vi "pulse_generator_multiheater_continuous_refnum.vi"(2 "Stop! Refnum":refnum<vi>, 3 "Pulse Generator Control Multiheater Refnums":T1) -> ()   [LabVIEW 2017]
uses:
  pulse_generator_controls_multiheater_refnums.ctl
  <vilib>/Utility/error.llb/DialogType.ctl
  <vilib>/DAQmx/write.llb/DAQmx Write (Digital 1D Bool NChan 1Samp 1Line).vi
  <vilib>/DAQmx/write.llb/DAQmx Write (Digital Wfm 1Chan NSamp).vi
  <vilib>/DAQmx/write.llb/DAQmx Write (Counter 1D Frequency 1Chan NSamp).vi
  <vilib>/DAQmx/read.llb/DAQmx Read (Counter DBL 1Chan 1Samp).vi
  <extravilib>/ChannelInstances/Stream-bool/Read With Abort.vi
  <extravilib>/ChannelInstances/Stream-bool/Write With Abort.vi
  <extravilib>/ChannelInstances/Stream-bool/EndpointRead.vi
  <extravilib>/ChannelInstances/Stream-bool/Endpoint.vi
  <vilib>/DAQmx/create/channels.llb/DAQmx Create Channel (CI-Position-Angular Encoder).vi
  <vilib>/DAQmx/create/channels.llb/DAQmx Create Channel (DO-Digital Output).vi
  <vilib>/DAQmx/configure/timing.llb/DAQmx Timing (Sample Clock).vi
  <vilib>/DAQmx/create/channels.llb/DAQmx Create Channel (CO-Pulse Generation-Frequency).vi
  <vilib>/DAQmx/configure/timing.llb/DAQmx Timing (Implicit).vi
  <vilib>/DAQmx/configure/trigger.llb/DAQmx Start Trigger (Digital Edge).vi
  <vilib>/Waveform/DWDTOps.llb/DWDT Uncompress Digital.vi
  <vilib>/DAQmx/miscellaneous.llb/DAQmx Fill In Error Info.vi
  <extravilib>/ChannelInstances/Stream-bool/Instantiate.vi
  <extravilib>/ChannelInstances/Stream-bool/)Channel.vi
  <resource>/ChannelSupport/_ChannelSupport/WaitIfNeeded.vi
  <extravilib>/ChannelInstances/Stream-bool.lvlib
  <resource>/objmgr/daqmx.rc
panel:
  out "Waveform Chart":dbl(graph)
  out "Stopped!":bool caption="OK"
  in  "Stop! Local":bool
  out "message":string
  in  "SwitchHelper":bool
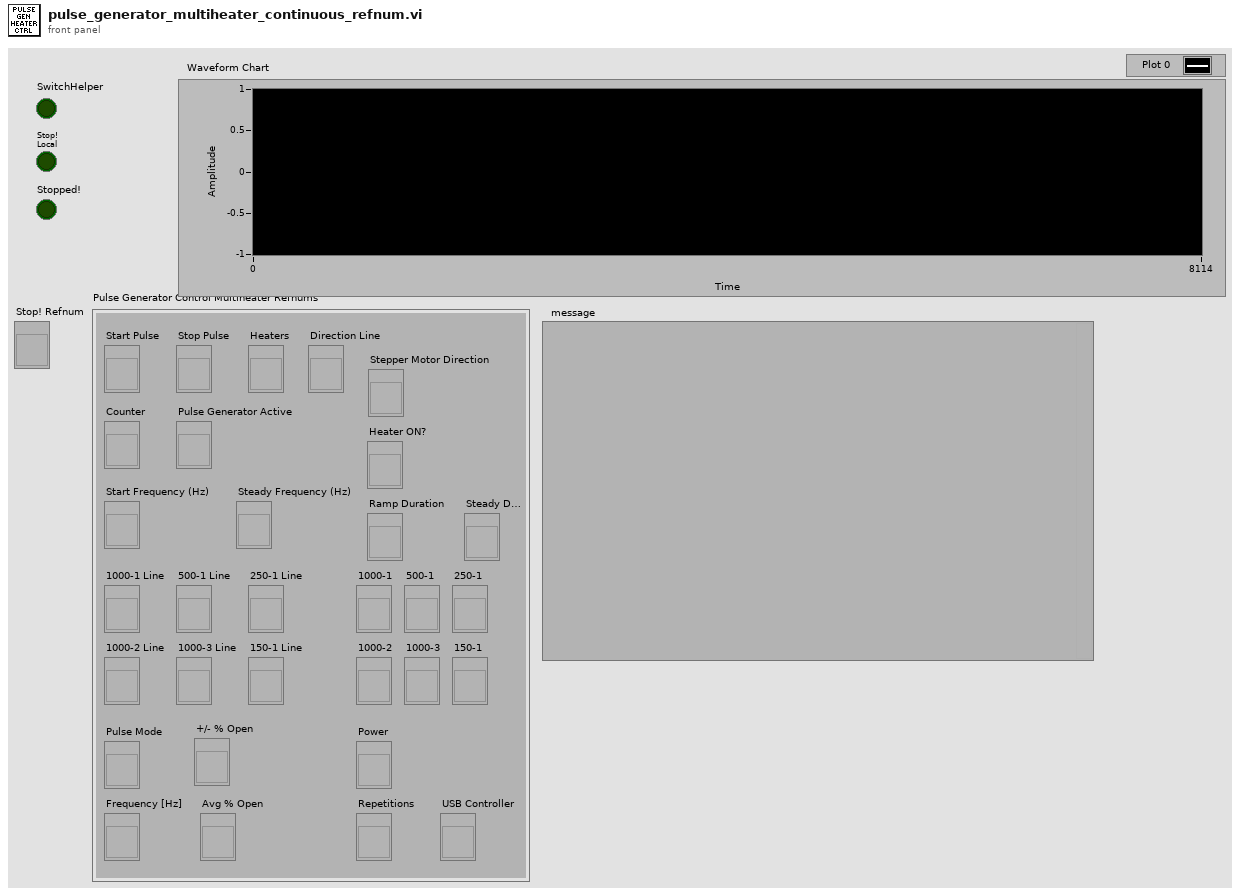
[diagram p1: front panel]
types:
  T1 = typedef "pulse_generator_controls_multiheater_refnums.ctl" = cluster{"Start Pulse":refnum<vi>, "Stop Pulse":refnum<vi>, "Heaters":refnum<vi>, "Counter":refnum<vi>, "Start Frequency (Hz)":refnum<vi>, "Pulse Generator Active":refnum<vi>, "Stepper Motor Direction":refnum<vi>, "Ramp Duration":refnum<vi>, "Direction Line":refnum<vi>, "1000-1 Line":refnum<vi>, "1000-2 Line":refnum<vi>, "1000-3 Line":refnum<vi>, "500-1 Line":refnum<vi>, "250-1 Line":refnum<vi>, "1000-1":refnum<vi>, "1000-2":refnum<vi>, "1000-3":refnum<vi>, "500-1":refnum<vi>, "250-1":refnum<vi>, "150-1":refnum<vi>, "Heater ON?":refnum<vi>, "150-1 Line":refnum<vi>, "Power":refnum<vi>, "Steady Frequency (Hz)":refnum<vi>, "Steady Duration ":refnum<vi>, "Pulse Mode":refnum<vi>, "Frequency [Hz]":refnum<vi>, "Avg % Open":refnum<vi>, "Repetitions":refnum<vi>, "+/- % Open":refnum<vi>, "USB Controller":refnum<vi>}
  T2 = enum8{"Enabled", "Disabled", "Disabled and Grayed Out"}
  T3 = typedef "DialogType.ctl" = u16
  T4 = cluster{"1000-1":refnum<vi>, "1000-2":refnum<vi>, "1000-3":refnum<vi>, "500-1":refnum<vi>, "250-1":refnum<vi>, "150-1":refnum<vi>}
  T5 = cluster{"1000-1 Line":refnum<vi>, "1000-2 Line":refnum<vi>, "1000-3 Line":refnum<vi>, "500-1 Line":refnum<vi>, "250-1 Line":refnum<vi>, "150-1 Line":refnum<vi>}
  T6 = typedef "Stream-bool.lvlib/)Channel.ctl" = refnum<queue>
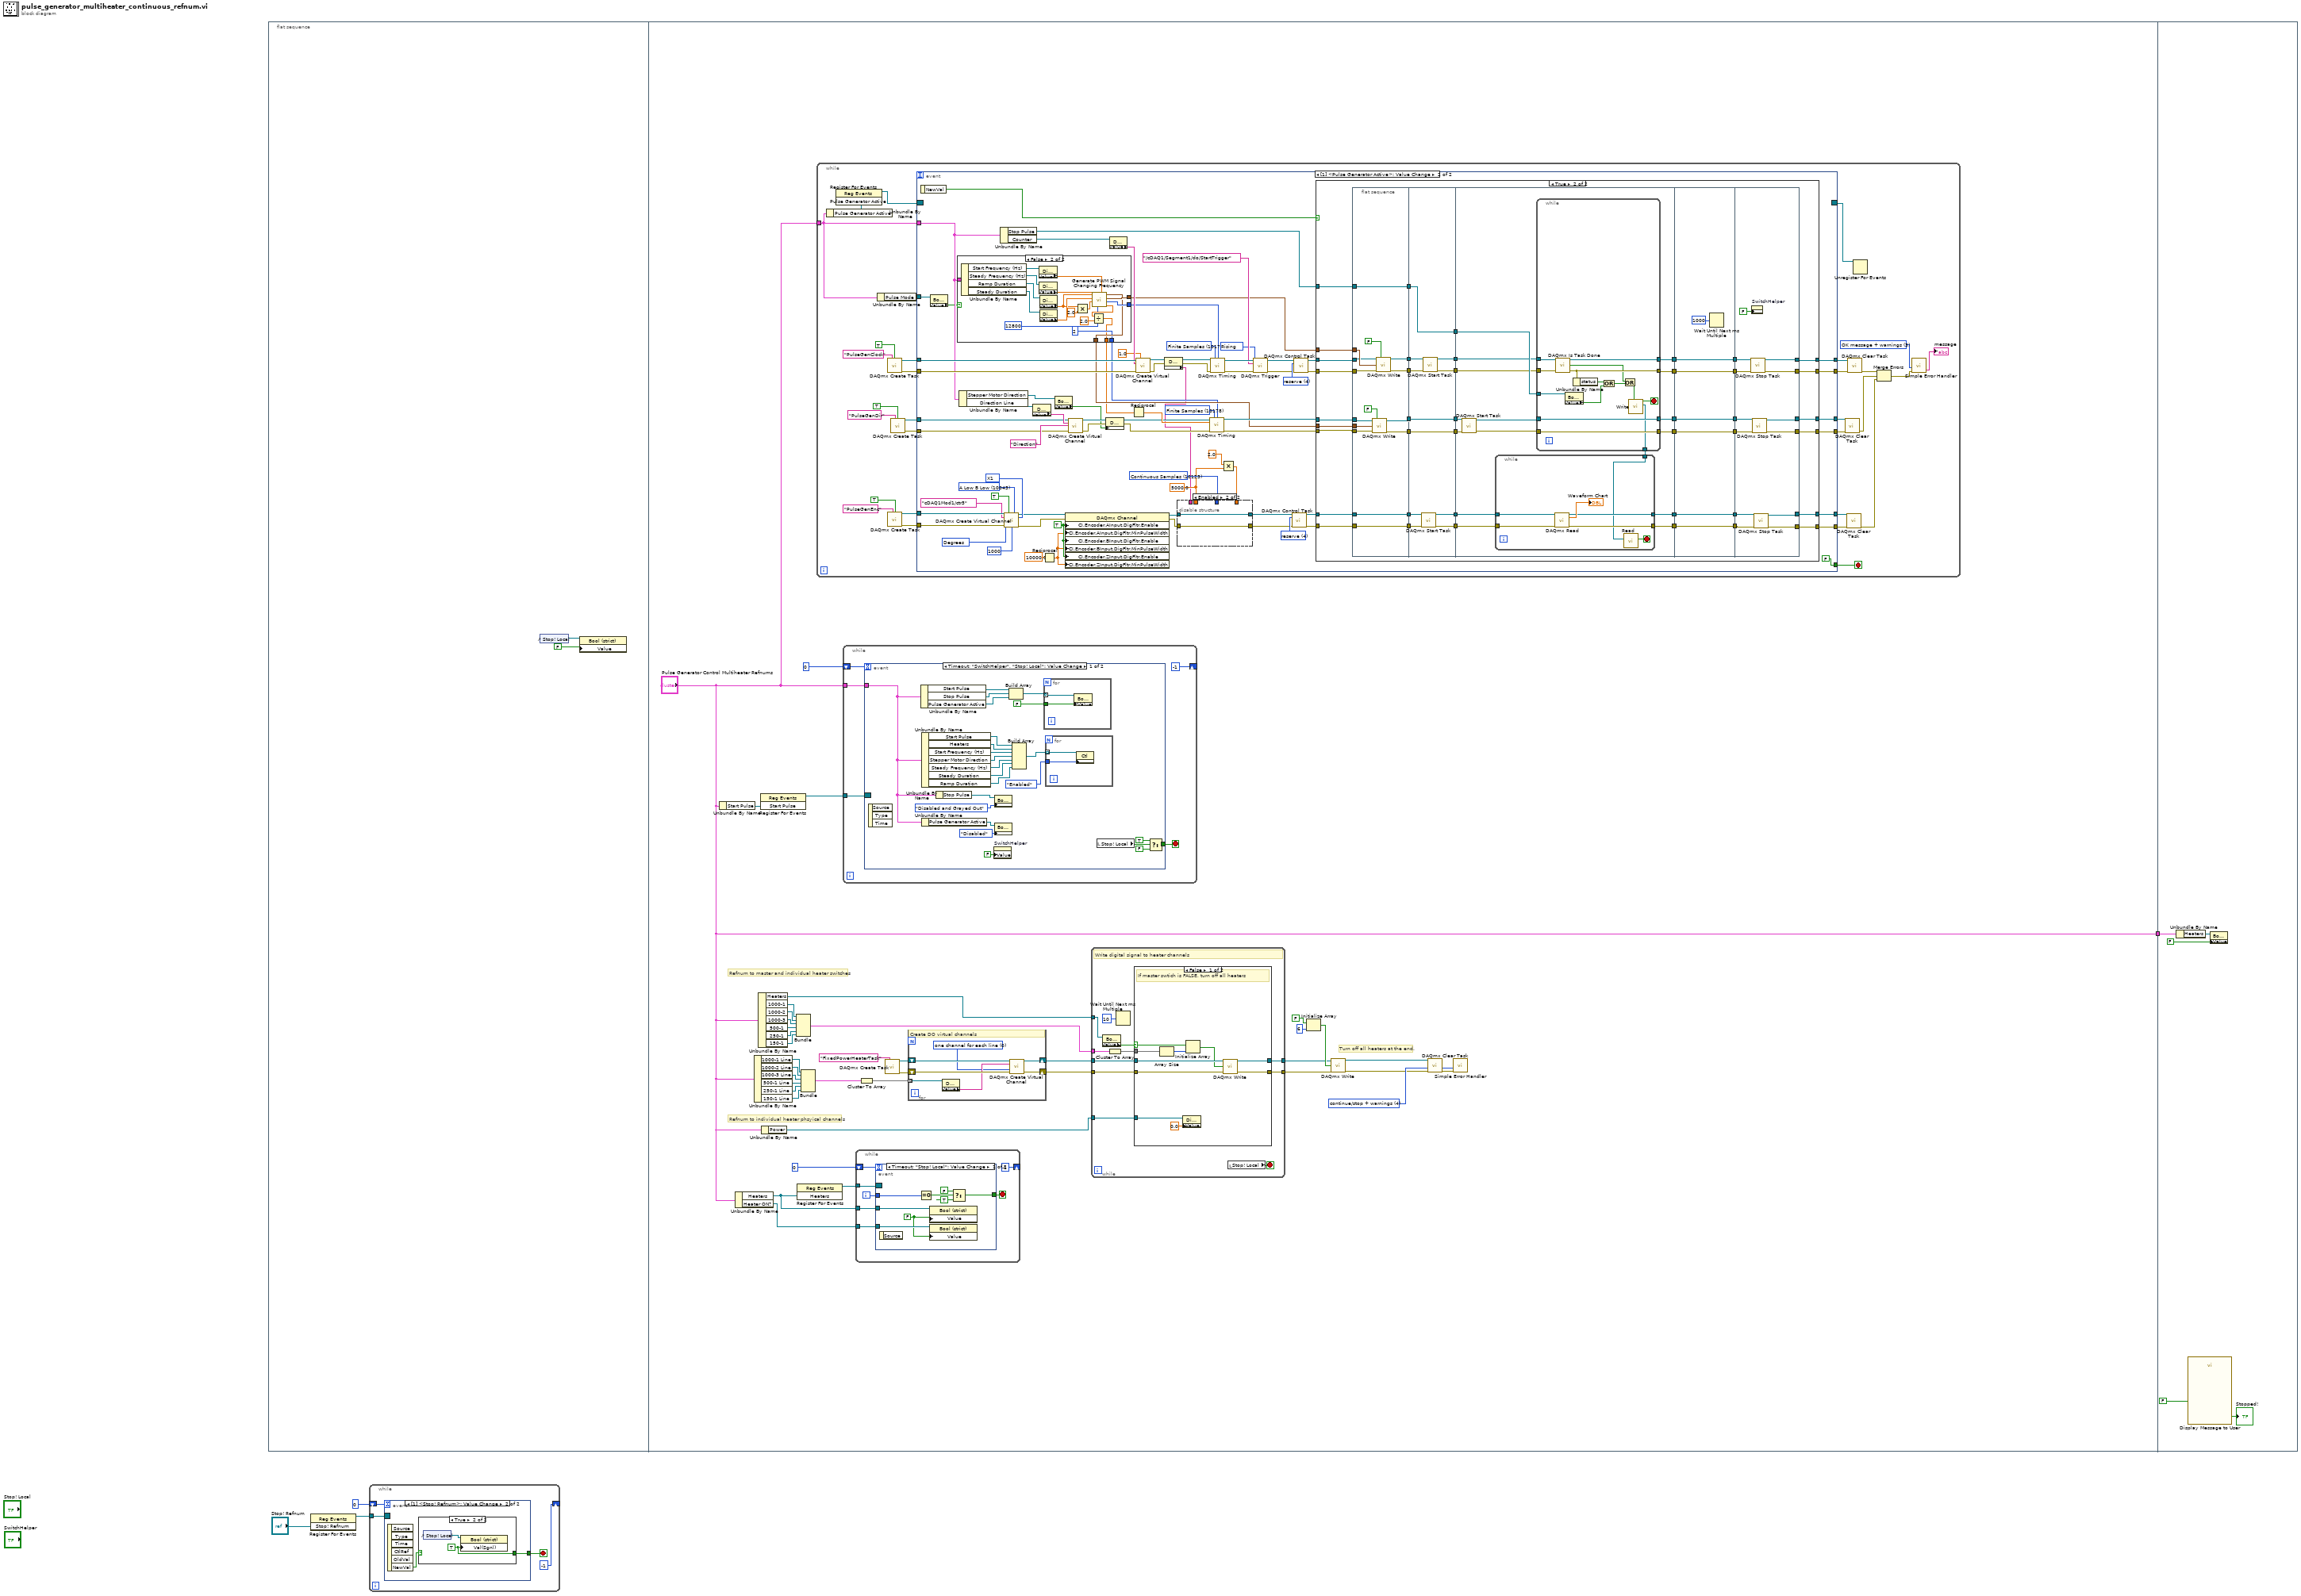
[diagram p0: block diagram]
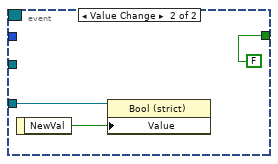
[diagram p2: hidden frame]
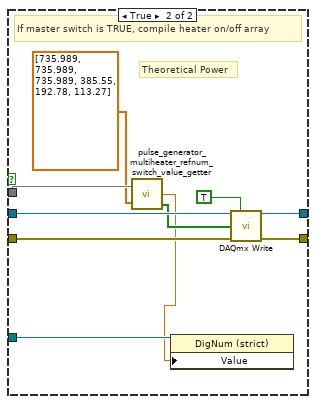
[diagram p3: hidden frame]
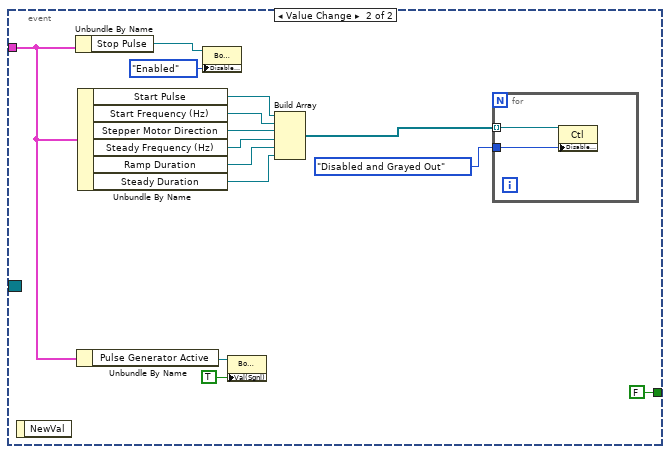
[diagram p4: hidden frame]
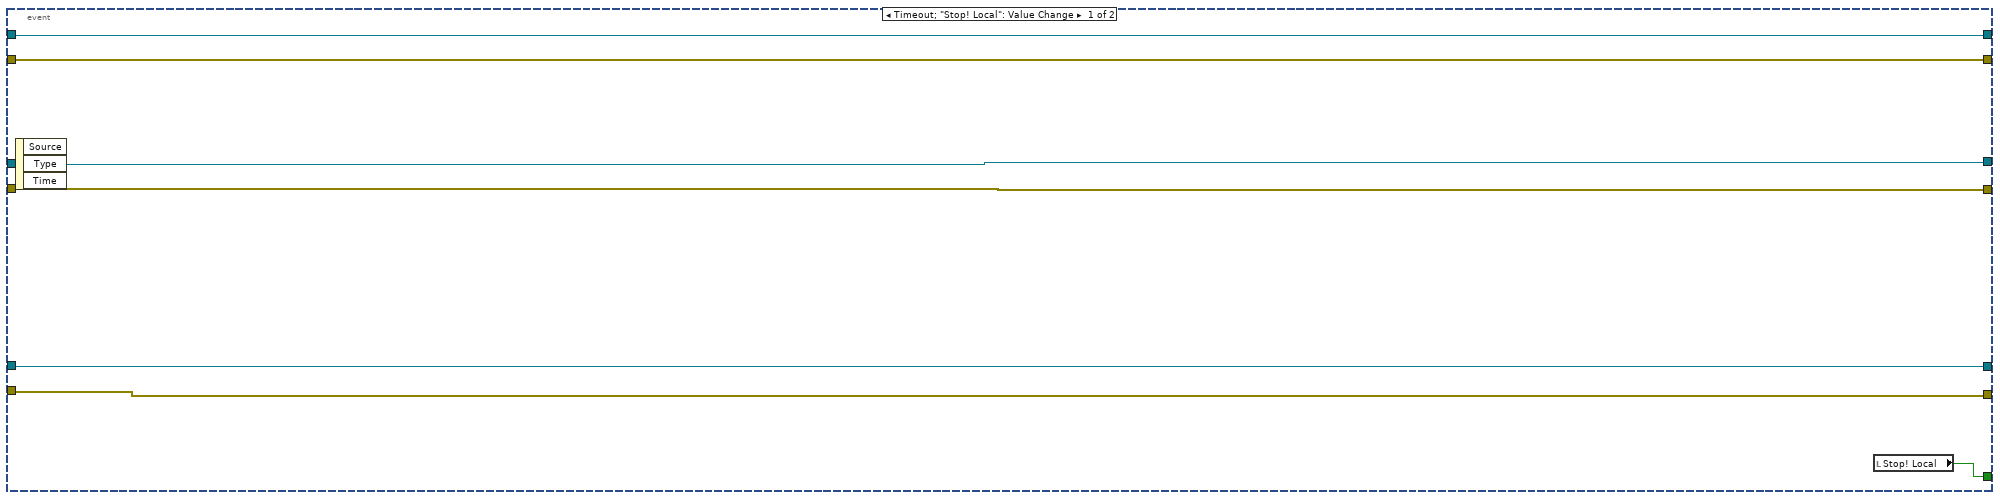
[diagram p5: hidden frame]
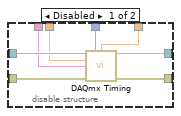
[diagram p6: hidden frame]
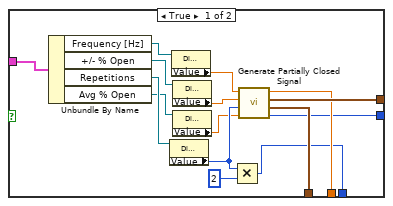
[diagram p7: hidden frame]
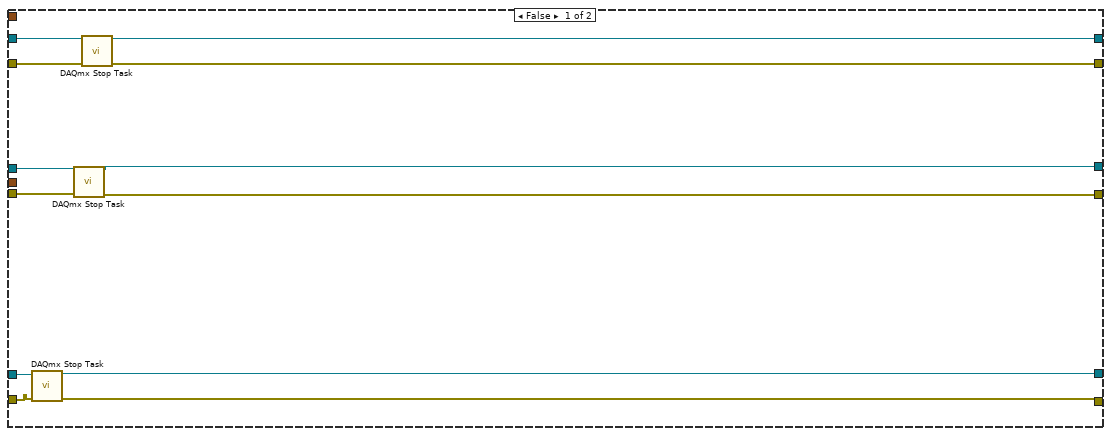
[diagram p8: hidden frame]
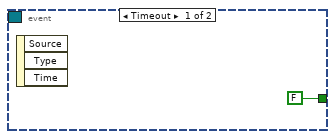
[diagram p9: hidden frame]
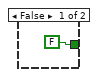
[diagram p10: hidden frame]
diagram:
  n1 = flat-sequence {
    tunnel: ["Pulse Generator Control Multiheater Refnums"] -> w1
    tunnel: w1 -> [w445]
    frame #0 {
      n2 = control-ref of="Stop! Local"() -> (w5:refnum<vi>)
      n3 = property class="Bool (strict)"(reference=w5, "Value"=FALSE) -> ()  [unwired: 1 in, 2 out]
    }
    frame #1 {
      w40 = T3 4 items=["no dialog", "OK message", "continue or stop message", "OK message + warnings", "continue/stop + warnings"] ("type of dialog (OK msg:1)")
      # "Turn off all heaters at the end."
      # "Refnum to individual heater phsyical channels"
      # "Refnum to master and individual heater switches"
      n4 = Unbundle By Name("Pulse Generator Control Multiheater Refnums") -> ("Start Pulse"=w43:refnum<vi>)
      n5 = Unbundle By Name("Pulse Generator Control Multiheater Refnums") -> ("Heaters"=w35:refnum<vi>, "Heater ON?"=w17:refnum<vi>)
      n6 = Unbundle By Name("Pulse Generator Control Multiheater Refnums") -> ("1000-1 Line"=w14:refnum<vi>, "1000-2 Line"=w13:refnum<vi>, "1000-3 Line"=w12:refnum<vi>, "500-1 Line"=w11:refnum<vi>, "250-1 Line"=w10:refnum<vi>, "150-1 Line"=w9:refnum<vi>)
      n7 = Unbundle By Name("Pulse Generator Control Multiheater Refnums") -> ("Heaters"=w34:refnum<vi>, "1000-1"=w33:refnum<vi>, "1000-2"=w32:refnum<vi>, "1000-3"=w31:refnum<vi>, "500-1"=w30:refnum<vi>, "250-1"=w28:refnum<vi>, "150-1"=w18:refnum<vi>)
      n8 = register-events(w43) -> (reference out=w44:refnum<event-registration>)  [unwired: 2 in, 1 out]
      n9 = Unbundle By Name("Pulse Generator Control Multiheater Refnums") -> ("Power"=w7:refnum<vi>)
      n10 = Bundle("1000-1"=w33, "1000-2"=w32, "1000-3"=w31, "500-1"=w30, "250-1"=w28, "150-1"=w18) -> (w15:T4)  [unwired: 1 in]
      n11 = register-events(w35) -> (reference out=w39:refnum<event-registration>)  [unwired: 2 in, 1 out]
      n12 = Bundle("1000-1 Line"=w14, "1000-2 Line"=w13, "1000-3 Line"=w12, "500-1 Line"=w11, "250-1 Line"=w10, "150-1 Line"=w9) -> (w16:T5)  [unwired: 1 in]
      n13 = while {
        tunnel: "Pulse Generator Control Multiheater Refnums" -> [w165]
        stop <- w173 stop-if-true
        w176 = T3 3 items=["no dialog", "OK message", "continue or stop message", "OK message + warnings", "continue/stop + warnings"] ("type of dialog (OK msg:1)")
        n14 = Unbundle By Name(w165) -> ("Pulse Generator Active"=w166:refnum<vi>)
        n15 = register-events(w166) -> (reference out=w178:refnum<event-registration>)  [unwired: 2 in, 1 out]
        n16 = Unbundle By Name(w165) -> ("Pulse Mode"=w157:refnum<vi>)
        n17 = call <vilib>:"DAQmx Create Task.vi"("new task name"="PulseGenClock", "auto cleanup"=TRUE) -> ("task out"=w175:refnum<k21>, "error out"=w174:errorcluster)  [unwired: 12 in]
        n18 = call <vilib>:"DAQmx Create Task.vi"("new task name"="PulseGenEnc", "auto cleanup"=TRUE) -> ("task out"=w159:refnum<k21>, "error out"=w158:errorcluster)  [unwired: 12 in]
        n19 = call <vilib>:"DAQmx Create Task.vi"("new task name"="PulseGenDir", "auto cleanup"=TRUE) -> ("task out"=w171:refnum<k21>, "error out"=w170:errorcluster)  [unwired: 12 in]
        n20 = event shown="[1] <Pulse Generator Active>: Value Change" {
          selector: w178 -> [_ _]
          dyn-events: [_ _] -> w164
          timeout: _ -> [_ _]
          tunnel: [w186 w247] -> w180
          tunnel: [w187 w246] -> w179
          tunnel: w175 -> [w187 w261]
          tunnel: w174 -> [w186 w260]
          tunnel: [w185 FALSE ("Stop! Local")] -> w173
          tunnel: w171 -> [w184 w257]
          tunnel: w170 -> [w183 w256]
          tunnel: [w184 w250] -> w163
          tunnel: [w183 w249] -> w162
          tunnel: w165 -> [_ w217]
          tunnel: w159 -> [w182 w234]
          tunnel: w158 -> [w181 w235]
          tunnel: [w182 w219] -> w155
          tunnel: [w181 w220] -> w156
          tunnel: w157 -> [_ w216]
          event Timeout; "Stop! Local": Value Change {
            n21 = event-data() -> ()  [unwired: 1 in, 3 out]
            n22 = local read "Stop! Local"() -> (w185:bool)
          }
          event Value Change {
            w228 = 10090 items=["X1"=10090, "X2"=10091, "X4"=10092, "Two Pulse Counting"=10313] ("decoding type")
            w189 = TRUE ("CI.Encoder.AInput.DigFltr.Enable")
            w195 = 10146 items=["Degrees"=10146, "Radians"=10273, "Ticks"=10304, "From Custom Scale"=10065] ("units")
            w206 = 10123 items=["Finite Samples"=10178, "Continuous Samples"=10123, "Hardware Timed Single Point"=12522] ("sample mode")
            w201 = 5000.0 ("rate")
            w221 = 10178 items=["Finite Samples"=10178, "Continuous Samples"=10123, "Hardware Timed Single Point"=12522] ("sample mode")
            w229 = 4 items=["verify"=2, "reserve"=4, "commit"=3, "unreserve"=5, "abort"=6] ("action")
            w231 = 10043 items=["A High B High"=10040, "A High B Low"=10041, "A Low B High"=10042, "A Low B Low"=10043] ("z index phase")
            w238 = 10280 items=["Rising"=10280, "Falling"=10171] ("edge")
            w245 = 4 items=["verify"=2, "reserve"=4, "commit"=3, "unreserve"=5, "abort"=6] ("action")
            w262 = 10178 items=["Finite Samples"=10178, "Continuous Samples"=10123, "Hardware Timed Single Point"=12522] ("sample mode")
            n23 = event-data() -> ("NewVal"=w263:bool)  [unwired: 1 in]
            n24 = property class="Bool (strict)"(reference=w216) -> ("Value"=w215:bool)  [unwired: 1 in, 2 out]
            n25 = case shown="False" w215 {
              tunnel: w217 -> [w288 w306]
              tunnel: [w282 w296] -> w236
              tunnel: [w279 w295] -> w214
              tunnel: [w281 w290] -> w203
              tunnel: [w280 w294] -> w207
              tunnel: [w276 2 ("Number of Samples")] -> w205
              frame True {
                n26 = Unbundle By Name(w288) -> ("Frequency [Hz]"=w287:refnum<vi>, "+/- % Open"=w286:refnum<vi>, "Repetitions"=w285:refnum<vi>, "Avg % Open"=w275:refnum<vi>)
                n27 = property class="DigNum (strict)"(reference=w285) -> ("Value"=w278:u32)  [unwired: 1 in, 2 out]
                n28 = property class="DigNum (strict)"(reference=w287) -> ("Value"=w284:dbl)  [unwired: 1 in, 2 out]
                n29 = property class="DigNum (strict)"(reference=w286) -> ("Value"=w283:dbl)  [unwired: 1 in, 2 out]
                n30 = property class="DigNum (strict)"(reference=w275) -> ("Value"=w274:dbl)  [unwired: 1 in, 2 out]
                n31 = Multiply(x=w278, y=u32 2) -> (x*y=w276:u32)
                n32 = call "Generate Partially Closed Signal.vi"("Avg % Open"=w274, "Repetitions"=w278, "+/- % Open"=w283, "Frequency[Hz]"=w284) -> ("Total # of Frequency Samples"=w279:i32, "Digital Waveform Graph"=w280:digitalwaveform, "CO Frequency"=w282:cluster{"duty cycle":dbl, "frequency":dbl}[], "dt"=w281:dbl)  [unwired: 2 in, 1 out]
              }
              frame False {
                n33 = Unbundle By Name(w306) -> ("Start Frequency (Hz)"=w307:refnum<vi>, "Steady Frequency (Hz)"=w305:refnum<vi>, "Ramp Duration"=w304:refnum<vi>, "Steady Duration"=w302:refnum<vi>)
                n34 = property class="DigNum (strict)"(reference=w307) -> ("Value"=w297:dbl)  [unwired: 1 in, 2 out]
                n35 = property class="DigNum (strict)"(reference=w305) -> ("Value"=w303:dbl)  [unwired: 1 in, 2 out]
                n36 = property class="DigNum (strict)"(reference=w304) -> ("Value"=w299:dbl)  [unwired: 1 in, 2 out]
                n37 = property class="DigNum (strict)"(reference=w302) -> ("Value"=w301:dbl)  [unwired: 1 in, 2 out]
                n38 = Multiply(x=w299, y=2.0) -> (x*y=w300:dbl)
                n39 = call "Generate PWM Signal Changing Frequency.vi"("Frequency Min"=w297, "Pulses per Revolution"=12800, "Frequency Max"=w303, "Ramp Down Duration"=w300, "Constant Duration"=w301, "Ramp Up Duration"=w299) -> ("Total Duration"=w292:dbl, "Number of Samples"=w295:i32, "Frequency Duty Cycle Data"=w296:cluster{"duty cycle":dbl, "frequency":dbl}[], "Digital Waveform Graph"=w294:digitalwaveform)  [unwired: 2 in]
                n40 = Divide(x=w292, y=2.0) -> (x/y=w290:dbl)
              }
            }
            n41 = Unbundle By Name(w217) -> ("Stepper Motor Direction"=w244:refnum<vi>, "Direction Line"=w253:refnum<vi>)
            n42 = Unbundle By Name(w217) -> ("Stop Pulse"=w252:refnum<vi>, "Counter"=w218:refnum<vi>)
            n43 = call-poly <vilib>:"DAQmx Create Virtual Channel.vi"("task in"=w234, "z index enable"=TRUE, "z index phase"=w231, "counter"=tag "cDAQ1Mod1/ctr3", "decoding type"=w228, "units"=w195, "error in"=w235, "pulses per revolution"=u32 1000) -> ("task out"=w193:refnum<k21>, "error out"=w192:errorcluster)  [unwired: 6 in]
            n44 = property class="DAQmxName"(reference=w253) -> ("Value"=w259:string)  [unwired: 1 in, 2 out]
            n45 = Reciprocal(x=10000.0) -> (1/x=w188:dbl)
            n46 = property class="Bool (strict)"(reference=w244) -> ("Value"=w208:bool)  [unwired: 1 in, 2 out]
            n47 = property class="DAQmx Channel"(reference=w193, error in=w192, "CI.Encoder.AInput.DigFltr.Enable"=w189, "CI.Encoder.AInput.DigFltr.MinPulseWidth"=w188, "CI.Encoder.BInput.DigFltr.Enable"=w189, "CI.Encoder.BInput.DigFltr.MinPulseWidth"=w188, "CI.Encoder.ZInput.DigFltr.Enable"=w189, "CI.Encoder.ZInput.DigFltr.MinPulseWidth"=w188) -> (reference out=w191:refnum<k21>, error out=w190:errorcluster)
            n48 = call-poly <vilib>:"DAQmx Create Virtual Channel.vi"("task in"=w257, "lines"=w259, "name to assign"="Direction", "error in"=w256) -> ("task out"=w212:refnum<k21>, "error out"=w210:errorcluster)  [unwired: 10 in]
            n49 = property class="DAQmx Channel"(reference=w212, error in=w210, "DO.InvertLines"=w208) -> (reference out=w211:refnum<k21>, error out=w209:errorcluster)
            n50 = property class="DAQmxName"(reference=w218) -> ("Value"=w251:string)  [unwired: 1 in, 2 out]
            n51 = Reciprocal(x=w203) -> (1/x=w213:dbl)
            n52 = call-poly <vilib>:"DAQmx Create Virtual Channel.vi"("task in"=w261, "frequency"=1.0, "counter"=w251, "error in"=w260) -> ("task out"=w200:refnum<k21>, "error out"=w198:errorcluster)  [unwired: 10 in]
            n53 = property class="DAQmx Channel"(reference=w200, error in=w198) -> (reference out=w199:refnum<k21>, error out=w197:errorcluster, "CO.CtrTimebaseSrc"=w196:tag)
            n54 = call-poly <vilib>:"DAQmx Timing.vi"("task/channels in"=w211, "sample mode"=w221, "samples per channel"=w205, "rate"=w213, "error in"=w209) -> ("task out"=w225:refnum<k21>, "error out"=w224:errorcluster)  [unwired: 9 in]
            n55 = call-poly <vilib>:"DAQmx Timing.vi"("task/channels in"=w199, "sample mode"=w262, "samples per channel"=w214, "error in"=w197) -> ("task out"=w243:refnum<k21>, "error out"=w242:errorcluster)  [unwired: 10 in]
            n56 = Multiply(x=2.0 ("y"), y=w201) -> (x*y=w204:dbl)
            n57 = disable-structure shown="Enabled" {
              disable-tunnel: w191 -> [w271 w273]
              disable-tunnel: w190 -> [w270 w272]
              disable-tunnel: [w269 w272] -> w223
              disable-tunnel: [w268 w273] -> w222
              disable-tunnel: w206 -> [w267 _]
              disable-tunnel: w204 -> [w266 _]
              disable-tunnel: w201 -> [w265 _]
              disable-tunnel: w196 -> [w264 _]
              frame Disabled {
                n58 = call-poly <vilib>:"DAQmx Timing.vi"("task/channels in"=w271, "sample mode"=w267, "samples per channel"=w266, "rate"=w265, "source"=w264, "error in"=w270) -> ("task out"=w268:refnum<k21>, "error out"=w269:errorcluster)  [unwired: 8 in]
              }
              frame Enabled {
              }
            }
            n59 = call-poly <vilib>:"DAQmx Trigger.vi"("task/channels in"=w243, "source"=tag "/cDAQ1/Segment1/do/StartTrigger" ("Start.DigEdge.Src"), "edge"=w238, "error in"=w242) -> ("task out"=w241:refnum<k21>, "error out"=w240:errorcluster)  [unwired: 10 in]
            n60 = call <vilib>:"DAQmx Control Task.vi"("task/channels in"=w222, "action"=w229, "error in"=w223) -> ("task out"=w227:refnum<k21>, "error out"=w226:errorcluster)  [unwired: 11 in]
            n61 = call <vilib>:"DAQmx Control Task.vi"("task/channels in"=w241, "action"=w245, "error in"=w240) -> ("task out"=w254:refnum<k21>, "error out"=w255:errorcluster)  [unwired: 11 in]
            n62 = case shown="True" w263 {
              tunnel: w254 -> [w319 w358]
              tunnel: w255 -> [w318 w353]
              tunnel: [w316 w360] -> w246
              tunnel: [w317 w359] -> w247
              tunnel: w252 -> [_ w357]
              tunnel: w225 -> [w315 w356]
              tunnel: w224 -> [w314 w352]
              tunnel: [w312 w355] -> w250
              tunnel: [w313 w354] -> w249
              tunnel: w236 -> [_ w351]
              tunnel: w227 -> [w311 w340]
              tunnel: w226 -> [w310 w339]
              tunnel: [w308 w333] -> w219
              tunnel: [w309 w334] -> w220
              tunnel: w207 -> [_ w332]
              frame False {
                n63 = call <vilib>:"DAQmx Stop Task.vi"("task/channels in"=w311, "error in"=w310) -> ("task out"=w308:refnum<k21>, "error out"=w309:errorcluster)  [unwired: 12 in]
                n64 = call <vilib>:"DAQmx Stop Task.vi"("task/channels in"=w315, "error in"=w314) -> ("task out"=w312:refnum<k21>, "error out"=w313:errorcluster)  [unwired: 12 in]
                n65 = call <vilib>:"DAQmx Stop Task.vi"("task/channels in"=w319, "error in"=w318) -> ("task out"=w316:refnum<k21>, "error out"=w317:errorcluster)  [unwired: 12 in]
              }
              frame True {
                n66 = flat-sequence {
                  tunnel: w356 -> [w374]
                  tunnel: w357 -> [w375]
                  tunnel: w358 -> [w368]
                  tunnel: w353 -> [w367]
                  tunnel: [w375] -> w350
                  tunnel: [w371] -> w348
                  tunnel: [w372] -> w347
                  tunnel: w352 -> [w373]
                  tunnel: w351 -> [w369]
                  tunnel: [w366] -> w345
                  tunnel: [w365] -> w344
                  tunnel: w340 -> [w363]
                  tunnel: w339 -> [w362]
                  tunnel: [w363] -> w338
                  tunnel: [w362] -> w337
                  tunnel: w332 -> [w361]
                  tunnel: w350 -> [w386]
                  tunnel: [w386] -> w349
                  tunnel: w348 -> [w380]
                  tunnel: w347 -> [w381]
                  tunnel: [w381] -> w346
                  tunnel: w345 -> [w385]
                  tunnel: w344 -> [w384]
                  tunnel: [w382] -> w343
                  tunnel: [w380] -> w342
                  tunnel: [w383] -> w341
                  tunnel: w338 -> [w379]
                  tunnel: w337 -> [w378]
                  tunnel: [w377] -> w336
                  tunnel: [w376] -> w335
                  tunnel: [w402] -> w331
                  tunnel: [w396] -> w329
                  tunnel: w349 -> [w400]
                  tunnel: [w397] -> w327
                  tunnel: [w401] -> w325
                  tunnel: w346 -> [w394]
                  tunnel: w343 -> [w398]
                  tunnel: w342 -> [w395]
                  tunnel: w341 -> [w399]
                  tunnel: w336 -> [w391]
                  tunnel: w335 -> [w390]
                  tunnel: [w388] -> w323
                  tunnel: [w389] -> w321
                  tunnel: w331 -> [w429]
                  tunnel: [w429] -> w330
                  tunnel: w329 -> [w428]
                  tunnel: [w428] -> w328
                  tunnel: w327 -> [w427]
                  tunnel: [w427] -> w326
                  tunnel: w325 -> [w426]
                  tunnel: [w426] -> w324
                  tunnel: w323 -> [w425]
                  tunnel: [w425] -> w322
                  tunnel: w321 -> [w424]
                  tunnel: [w424] -> w320
                  tunnel: [w439] -> w359
                  tunnel: [w440] -> w360
                  tunnel: w330 -> [w441]
                  tunnel: [w435] -> w355
                  tunnel: w328 -> [w436]
                  tunnel: [w434] -> w354
                  tunnel: w326 -> [w437]
                  tunnel: w324 -> [w438]
                  tunnel: w322 -> [w431]
                  tunnel: w320 -> [w430]
                  tunnel: [w432] -> w333
                  tunnel: [w433] -> w334
                  frame #0 {
                    n67 = call-poly <vilib>:"DAQmx Write.vi"("task/channels in"=w374, "auto start"=FALSE, "data"=w361, "error in"=w373) -> ("task out"=w372:refnum<k21>, "error out"=w371:errorcluster)  [unwired: 9 in, 1 out]
                    n68 = call-poly <vilib>:"DAQmx Write.vi"("task/channels in"=w368, "auto start"=FALSE, "data"=w369, "error in"=w367) -> ("task out"=w366:refnum<k21>, "error out"=w365:errorcluster)  [unwired: 9 in, 1 out]
                  }
                  frame #1 {
                    n69 = call <vilib>:"DAQmx Start Task.vi"("task/channels in"=w379, "error in"=w378) -> ("task out"=w377:refnum<k21>, "error out"=w376:errorcluster)  [unwired: 12 in]
                    n70 = call <vilib>:"DAQmx Start Task.vi"("task/channels in"=w385, "error in"=w384) -> ("task out"=w382:refnum<k21>, "error out"=w383:errorcluster)  [unwired: 12 in]
                  }
                  frame #2 {
                    n71 = call <vilib>:"DAQmx Start Task.vi"("task/channels in"=w394, "error in"=w395) -> ("task out"=w393:refnum<k21>, "error out"=w392:errorcluster)  [unwired: 12 in]
                    n72 = while {
                      tunnel: w399 -> [w421]
                      tunnel: w398 -> [w422]
                      tunnel: [w413] -> w402
                      tunnel: [w419] -> w401
                      tunnel: w400 -> [w415]
                      tunnel: w393 -> [w412]
                      tunnel: w392 -> [w411]
                      tunnel: [w412] -> w397
                      tunnel: [w411] -> w396
                      tunnel: [w410] -> w387
                      stop <- w417 stop-if-true
                      n73 = call <vilib>:"DAQmx Is Task Done.vi"("task/channels in"=w422, "error in"=w421) -> ("task out"=w413:refnum<k21>, "task done?"=w416:bool, "error out"=w419:errorcluster)  [unwired: 11 in]
                      n74 = property class="Bool (strict)"(reference=w415) -> ("Value"=w414:bool)  [unwired: 1 in, 2 out]
                      n75 = Unbundle By Name(w419) -> ("status"=w420:bool)
                      n76 = Or(x=w420, y=w414) -> (x .or. y?=w418:bool)
                      n77 = Or(x=w416, y=w418) -> (x .or. y?=w417:bool)
                      n78 = call <extravilib>:"Write.vi"("element"=w417) -> ("channel"=w410:T6)  [unwired: 8 in, 2 out]
                    }
                    n79 = while {
                      tunnel: w391 -> [w408]
                      tunnel: w390 -> [w407]
                      tunnel: [w406] -> w389
                      tunnel: [w405] -> w388
                      tunnel: w387 -> [w404]
                      stop <- w403 stop-if-true
                      n80 = call-poly <vilib>:"DAQmx Read.vi"("task/channels in"=w408, "error in"=w407) -> ("task out"=w405:refnum<k21>, "data"=→"Waveform Chart":dbl, "error out"=w406:errorcluster)  [unwired: 11 in]
                      n81 = call <extravilib>:"Read.vi"("channel"=w404) -> ("element"=w403:bool)  [unwired: 6 in, 4 out]
                    }
                  }
                  frame #3 {
                    n82 = Wait Until Next ms Multiple(millisecond multiple=u32 1000) -> ()  [unwired: 1 out]
                  }
                  frame #4 {
                    n83 = call <vilib>:"DAQmx Stop Task.vi"("task/channels in"=w441, "error in"=w438) -> ("task out"=w440:refnum<k21>, "error out"=w439:errorcluster)  [unwired: 12 in]
                    n84 = property on="SwitchHelper" class="Bool (strict)"("Val(Sgnl)"=FALSE ("Value (Signaling)")) -> ()  [unwired: 2 in, 2 out]
                    n85 = call <vilib>:"DAQmx Stop Task.vi"("task/channels in"=w437, "error in"=w436) -> ("task out"=w435:refnum<k21>, "error out"=w434:errorcluster)  [unwired: 12 in]
                    n86 = call <vilib>:"DAQmx Stop Task.vi"("task/channels in"=w431, "error in"=w430) -> ("task out"=w432:refnum<k21>, "error out"=w433:errorcluster)  [unwired: 12 in]
                  }
                }
              }
            }
          }
        }
        n87 = call <vilib>:"DAQmx Clear Task.vi"("task in"=w163, "error in"=w162) -> ("error out"=w153:errorcluster)  [unwired: 13 in]
        n88 = call <vilib>:"DAQmx Clear Task.vi"("task in"=w155, "error in"=w156) -> ("error out"=w152:errorcluster)  [unwired: 13 in]
        n89 = call <vilib>:"DAQmx Clear Task.vi"("task in"=w179, "error in"=w180) -> ("error out"=w154:errorcluster)  [unwired: 13 in]
        n90 = Unregister For Events(event registration refnum=w164) -> ()  [unwired: 1 in, 1 out]
        n91 = Merge Errors(w154, w153, w152) -> (w151:errorcluster)
        n92 = call <vilib>:"Simple Error Handler.vi"("type of dialog (OK msg:1)"=w176, "error in (no error)"=w151) -> ("message"=→"message":string)  [unwired: 3 in, 4 out]
      }
      n93 = while {
        shift-right: [-1] -> _
        shift-left: 0 -> [w106]
        tunnel: w44 -> [w104]
        tunnel: "Pulse Generator Control Multiheater Refnums" -> [w102]
        stop <- w103 stop-if-true
        n94 = event shown="[0] Timeout;  \"SwitchHelper\", \"Stop! Local\": Value Change" {
          selector: w104 -> [_ _]
          dyn-events: _ -> [_ _]
          timeout: w106 -> [_ _]
          tunnel: [w127 FALSE ("Value")] -> w103
          tunnel: w102 -> [w109 w137]
          event Timeout; "SwitchHelper", "Stop! Local": Value Change {
            n95 = event-data() -> ()  [unwired: 1 in, 3 out]
            n96 = Unbundle By Name(w109) -> ("Start Pulse"=w116:refnum<vi>, "Stop Pulse"=w115:refnum<vi>, "Pulse Generator Active"=w114:refnum<vi>)
            n97 = Unbundle By Name(w109) -> ("Start Pulse"=w120:refnum<vi>, "Heaters"=w124:refnum<vi>, "Start Frequency (Hz)"=w123:refnum<vi>, "Stepper Motor Direction"=w122:refnum<vi>, "Steady Frequency (Hz)"=w121:refnum<vi>, "Steady Duration"=w108:refnum<vi>, "Ramp Duration"=w107:refnum<vi>)
            n98 = Unbundle By Name(w109) -> ("Pulse Generator Active"=w112:refnum<vi>)
            n99 = Unbundle By Name(w109) -> ("Stop Pulse"=w111:refnum<vi>)
            n100 = property on="SwitchHelper" class="Bool (strict)"("Value"=FALSE) -> ()  [unwired: 2 in, 2 out]
            n101 = property class="Bool (strict)"(reference=w111, "DisabledEnum"=T2."Disabled and Grayed Out" ("Disabled")) -> ()  [unwired: 1 in, 2 out]
            n102 = property class="Bool (strict)"(reference=w112, "DisabledEnum"=T2."Disabled" ("Disabled")) -> ()  [unwired: 1 in, 2 out]
            n103 = Build Array(w116, w115, w114) -> (w117:refnum<vi>[])
            n104 = Build Array(w120, w124, w123, w122, w121, w108, w107) -> (w119:refnum<vi>[])
            n105 = for {
              tunnel: w117 -> [w132] mode=indexing
              tunnel: FALSE ("Value") -> [w131]
              n106 = property class="Bool (strict)"(reference=w132, "Value"=w131) -> ()  [unwired: 1 in, 2 out]
            }
            n107 = for {
              tunnel: w119 -> [w134] mode=indexing
              tunnel: T2."Enabled" ("Disabled") -> [w133]
              n108 = property class="Ctl"(reference=w134, "DisabledEnum"=w133) -> ()  [unwired: 1 in, 2 out]
            }
            n109 = local read "Stop! Local"() -> (w128:bool)
            n110 = Select(t=TRUE ("Value"), s=w128, f=FALSE ("Value")) -> (s? t:f=w127:bool)
          }
          event Value Change {
            n111 = event-data() -> ()  [unwired: 1 in, 1 out]
            n112 = Unbundle By Name(w137) -> ("Stop Pulse"=w141:refnum<vi>)
            n113 = Unbundle By Name(w137) -> ("Pulse Generator Active"=w139:refnum<vi>)
            n114 = Unbundle By Name(w137) -> ("Start Pulse"=w144:refnum<vi>, "Start Frequency (Hz)"=w145:refnum<vi>, "Stepper Motor Direction"=w146:refnum<vi>, "Steady Frequency (Hz)"=w147:refnum<vi>, "Ramp Duration"=w136:refnum<vi>, "Steady Duration"=w135:refnum<vi>)
            n115 = property class="Bool (strict)"(reference=w141, "DisabledEnum"=T2."Enabled" ("Disabled")) -> ()  [unwired: 1 in, 2 out]
            n116 = property class="Bool (strict)"(reference=w139, "Val(Sgnl)"=TRUE ("Value")) -> ()  [unwired: 1 in, 2 out]
            n117 = Build Array(w144, w145, w146, w147, w136, w135) -> (w143:refnum<vi>[])
            n118 = for {
              tunnel: w143 -> [w150] mode=indexing
              tunnel: T2."Disabled and Grayed Out" ("Disabled") -> [w149]
              n119 = property class="Ctl"(reference=w150, "DisabledEnum"=w149) -> ()  [unwired: 1 in, 2 out]
            }
          }
        }
      }
      n120 = while {
        tunnel: w39 -> [w59]
        shift-right: [-1 ("millisecond multiple")] -> _
        shift-left: 0 ("millisecond multiple") -> [w58]
        tunnel: w35 -> [w56]
        tunnel: w17 -> [w53]
        i -> [w55]
        stop <- w54 stop-if-true
        n121 = event shown="[0] Timeout;  \"Stop! Local\": Value Change" {
          selector: w59 -> [_ _]
          dyn-events: _ -> [_ _]
          timeout: w58 -> [_ _]
          tunnel: w56 -> [w67 _]
          tunnel: w55 -> [w65 _]
          tunnel: [w62 FALSE ("f")] -> w54
          tunnel: w53 -> [w61 w68]
          event Timeout; "Stop! Local": Value Change {
            w60 = FALSE ("Value")
            n122 = event-data() -> ()  [unwired: 1 in, 1 out]
            n123 = Equal To 0?(x=w65) -> (x = 0?=w66:bool)
            n124 = property class="Bool (strict)"(reference=w67, "Value"=w60) -> ()  [unwired: 1 in, 2 out]
            n125 = property class="Bool (strict)"(reference=w61, "Value"=w60) -> ()  [unwired: 1 in, 2 out]
            n126 = Select(t=FALSE, s=w66, f=TRUE) -> (s? t:f=w62:bool)
          }
          event Value Change {
            n127 = event-data() -> ("NewVal"=w69:bool)  [unwired: 1 in]
            n128 = property class="Bool (strict)"(reference=w68, "Value"=w69) -> ()  [unwired: 1 in, 2 out]
          }
        }
      }
      n129 = Cluster To Array(cluster=w16) -> (array=w29:refnum<vi>[])
      n130 = call <vilib>:"DAQmx Create Task.vi"("new task name"="FixedPowerHeaterTask") -> ("task out"=w38:refnum<k21>, "error out"=w37:errorcluster)  [unwired: 13 in]
      n131 = for {
        tunnel: w29 -> [w48] mode=indexing
        shift-right: [w52] -> w21
        shift-left: w38 -> [w50]
        shift-right: [w51] -> w20
        shift-left: w37 -> [w49]
        w46 = 0 items=["one channel for each line", "one channel for all lines"] ("line grouping")
        # "Create DO virtual channels"
        n132 = property class="DAQmxName"(reference=w48) -> ("Value"=w47:string)  [unwired: 1 in, 2 out]
        n133 = call-poly <vilib>:"DAQmx Create Virtual Channel.vi"("task in"=w50, "lines"=w47, "line grouping"=w46, "error in"=w49) -> ("task out"=w52:refnum<k21>, "error out"=w51:errorcluster)  [unwired: 10 in]
      }
      n134 = while {
        tunnel: w21 -> [w79]
        tunnel: w20 -> [w78]
        tunnel: w34 -> [w75]
        tunnel: [w77] -> w23
        tunnel: [w76] -> w22
        tunnel: w15 -> [w73]
        tunnel: w7 -> [w71]
        stop <- w80 stop-if-true
        # "Write digital signal to heater channels"
        n135 = property class="Bool (strict)"(reference=w75) -> ("Value"=w74:bool)  [unwired: 1 in, 2 out]
        n136 = Cluster To Array(cluster=w73) -> (array=w72:refnum<vi>[])
        n137 = Wait Until Next ms Multiple(millisecond multiple=u32 10) -> ()  [unwired: 1 out]
        n138 = case shown="False" w74 {
          selector: w74 -> [w84 _]
          tunnel: w79 -> [w91 w100]
          tunnel: w78 -> [w90 w99]
          tunnel: [w88 w101] -> w77
          tunnel: [w89 w98] -> w76
          tunnel: w72 -> [w86 w96]
          tunnel: w71 -> [w83 w93]
          frame False {
            # "If master swtich is FALSE, turn off all heaters"
            n139 = Array Size(array=w86) -> (size(s)=w87:i32)
            n140 = property class="DigNum (strict)"(reference=w83, "Value"=0.0) -> ()  [unwired: 1 in, 2 out]
            n141 = Initialize Array(w84, w87) -> (w85:bool[])
            n142 = call-poly <vilib>:"DAQmx Write.vi"("task/channels in"=w91, "data"=w85, "error in"=w90) -> ("task out"=w88:refnum<k21>, "error out"=w89:errorcluster)  [unwired: 10 in, 1 out]
          }
          frame True {
            # "Theoretical Power"
            # "If master switch is TRUE, compile heater on/off array"
            n143 = call "pulse_generator_multiheater_refnum_switch_value_getter.vi"("On/Off Refnums"=w96, "Power Array"=dbl[] [735.989, 735.989, 735.989, 385.55, 192.78, 113.27]) -> ("Total Power"=w92:dbl, "Digital"=w95:bool[])  [unwired: 1 out]
            n144 = property class="DigNum (strict)"(reference=w93, "Value"=w92) -> ()  [unwired: 1 in, 2 out]
            n145 = call-poly <vilib>:"DAQmx Write.vi"("task/channels in"=w100, "auto start"=TRUE, "data"=w95, "error in"=w99) -> ("task out"=w101:refnum<k21>, "error out"=w98:errorcluster)  [unwired: 9 in, 1 out]
          }
        }
        n146 = local read "Stop! Local"() -> (w80:bool)
      }
      n147 = Initialize Array(FALSE ("element"), 6 ("dimension size")) -> (w24:bool[])
      n148 = call-poly <vilib>:"DAQmx Write.vi"("task/channels in"=w23, "data"=w24, "error in"=w22) -> ("task out"=w27:refnum<k21>, "error out"=w26:errorcluster)  [unwired: 10 in, 1 out]
      n149 = call <vilib>:"DAQmx Clear Task.vi"("task in"=w27, "error in"=w26) -> ("error out"=w42:errorcluster)  [unwired: 13 in]
      n150 = call <vilib>:"Simple Error Handler.vi"("type of dialog (OK msg:1)"=w40, "error in (no error)"=w42) -> ()  [unwired: 3 in, 5 out]
    }
    frame #2 {
      n151 = Unbundle By Name(w445) -> ("Heaters"=w444:refnum<vi>)
      n152 = call "Display Message to User"("Enable"=FALSE) -> ("OK"=→"Stopped!":bool)  [unwired: 9 in, 1 out]
      n153 = property class="Bool (strict)"(reference=w444, "Value"=FALSE) -> ()  [unwired: 1 in, 2 out]
    }
  }
  n154 = register-events("Stop! Refnum") -> (reference out=w3:refnum<event-registration>)  [unwired: 2 in, 1 out]
  n155 = while {
    tunnel: w3 -> [w451]
    shift-right: [-1] -> _
    shift-left: 0 -> [w450]
    stop <- w448 stop-if-true
    n156 = event shown="[1] <Stop! Refnum>: Value Change" {
      selector: w451 -> [_ _]
      dyn-events: _ -> [_ _]
      timeout: w450 -> [_ _]
      tunnel: [FALSE ("Value (Signaling)") w453] -> w448
      event Timeout {
        n157 = event-data() -> ()  [unwired: 1 in, 3 out]
      }
      event Value Change {
        n158 = event-data() -> ("NewVal"=w454:bool)  [unwired: 1 in, 5 out]
        n159 = case shown="True" w454 {
          tunnel: [FALSE ("Value (Signaling)") w457] -> w453
          frame False {
          }
          frame True {
            w457 = TRUE ("Value (Signaling)")
            n160 = control-ref of="Stop! Local"() -> (w456:refnum<vi>)
            n161 = property class="Bool (strict)"(reference=w456, "Val(Sgnl)"=w457) -> ()  [unwired: 1 in, 2 out]
          }
        }
      }
    }
  }
